vi "Queue Comms Dequeue.vi"(8 "error in (no error)":errorcluster, 10 "timeout in ms (-1)":i32) -> (0 "error out":errorcluster, 3 "element":T1={"Data"=variant, "Action"=enum."Init"})   [LabVIEW 2018, in "Controller (Host).lvlib"]
doc: "This subVI dequeues an element from the communications queue using the Queue Comms FGV"
uses:
  Controller (Host).lvlib
  Private Controls/Module Data.ctl
  Private Controls/Module Action.ctl
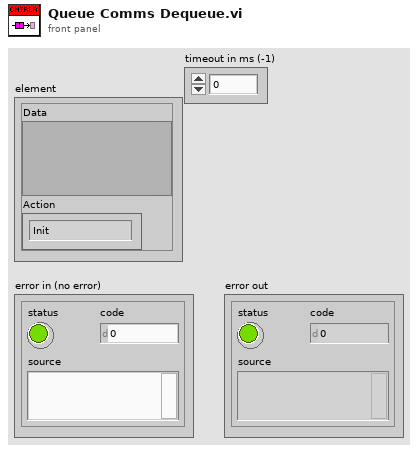
[diagram p1: front panel]
types:
  T1 = typedef "Controller (Host).lvlib/Module Data.ctl" = cluster{"Data":variant, "Action":T2}
  T2 = typedef "Controller (Host).lvlib/Module Action.ctl" = enum8{"Timeout", "New Data", "Value to Monitor", "Init", "Reset Dev_Min_Max", "Error", "Exit", "Prompt Test Info", "Update Test Info", "Prompt Variable Info", "Load APU Setup Data"}
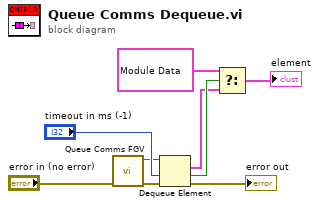
[diagram p0: block diagram]
diagram:
  n1 = call "Queue Comms FGV.vi"("error in (no error)"="error in (no error)") -> ("error out"=w2:errorcluster, "Queue out"=w3:refnum<queue>)  [unwired: 9 in]
  n2 = Dequeue Element(queue=w3, timeout in ms (-1)="timeout in ms (-1)", error in (no error)=w2) -> (element=w5:T1, timed out?=w6:bool, error out=→"error out":errorcluster)  [unwired: 1 out]
  n3 = Select(t=T1 {"Data"=variant, "Action"=enum."Timeout"}, s=w6, f=w5) -> (s? t:f=→"element":T1)
